vi "Comm EXE Set EXE Path.vi"(8 "error in (no error)":errorcluster, 10 "EXE Path":path, 11 "niDTS Comm EXE in":refnum<class "niDTS Comm EXE.lvclass">) -> (0 "error out":errorcluster, 3 "niDTS Comm EXE out":refnum<class "niDTS Comm EXE.lvclass">)   [LabVIEW 2015, in "niDTS CommLib.lvlib" / "niDTS Comm EXE.lvclass"]
uses:
  niDTS Comm EXE.lvclass
  niDTS Comm EXE.lvclass/niDTS Comm EXE.ctl
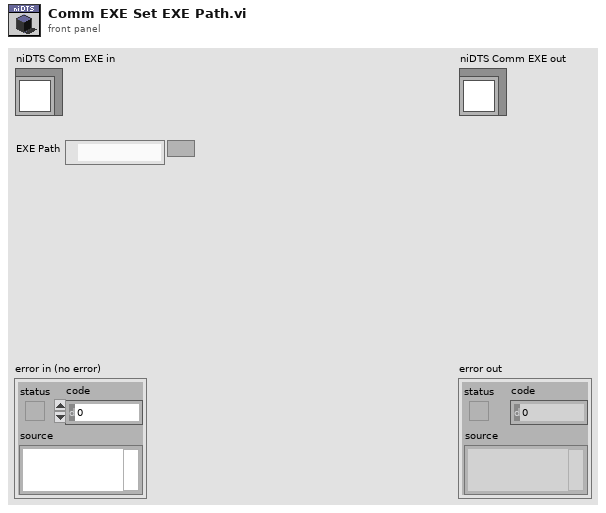
[diagram p1: front panel]
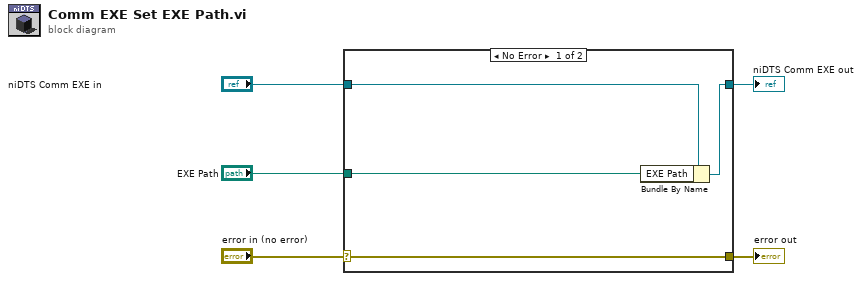
[diagram p0: block diagram]
diagram:
  n1 = case shown="No Error" "error in (no error)" {
    selector: "error in (no error)" -> [w9 w10]
    tunnel: [w9 w10] -> w4
    tunnel: [w7 w11] -> w2
    tunnel: "niDTS Comm EXE in" -> [w8 w11]
    tunnel: "EXE Path" -> [w6 _]
    frame No Error {
      n2 = Bundle By Name(cluster=w8, "EXE Path"=w6) -> (w7:refnum<class "niDTS Comm EXE.lvclass">)
    }
    frame Error {
    }
  }
  "error out" <- w4
  "niDTS Comm EXE out" <- w2
